vi "SetBox.vi"(8 "error in (no error)":errorcluster, 10 "Box":T1, 11 "FolloWin in":refnum<class "FolloWin.lvclass">) -> (0 "error out":errorcluster, 3 "FolloWin out":refnum<class "FolloWin.lvclass">)   [LabVIEW 2023, in "FolloWin.lvclass"]
doc: "Sets the box (in screen coordinates) \nThe Box defines the active area of FolloWin, meaning, it will only show the FolloWin window if your mouse cursor is inside the box's boundries."
uses:
  FolloWin.lvclass
  <vilib>/Utility/miscctls.llb/LVRectTypeDef.ctl
  FolloWin.lvclass/FolloWin.ctl
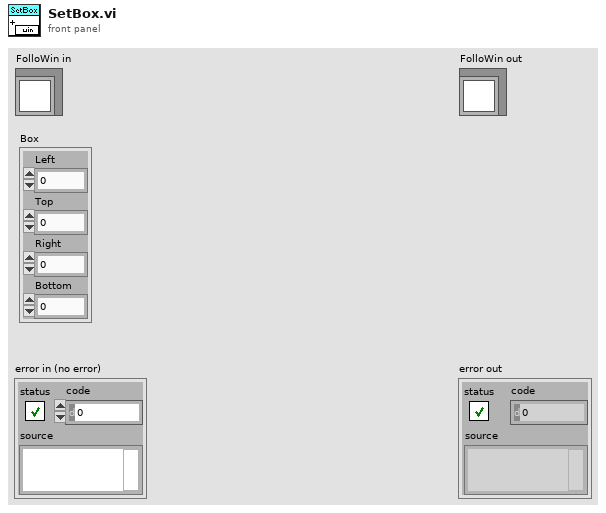
[diagram p1: front panel]
types:
  T1 = typedef "LVRectTypeDef.ctl" = cluster{"Left":i16, "Top":i16, "Right":i16, "Bottom":i16}
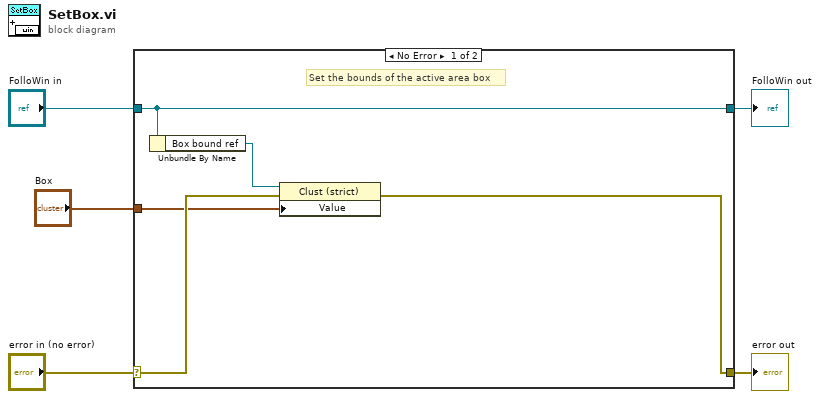
[diagram p0: block diagram]
diagram:
  n1 = case shown="No Error" "error in (no error)" {
    selector: "error in (no error)" -> [w8 w12]
    tunnel: [w7 w12] -> w4
    tunnel: [w10 w11] -> w2
    tunnel: "FolloWin in" -> [w10 w11]
    tunnel: "Box" -> [w6 _]
    frame No Error {
      # "Set the bounds of the active area box"
      n2 = Unbundle By Name(w10) -> ("Box bound ref"=w9:refnum<vi>)
      n3 = property on="Property Node" class="Clust (strict)"(reference=w9, error in=w8, "Value"=w6) -> (error out=w7:errorcluster)  [unwired: 1 out]
    }
    frame Error {
    }
  }
  "error out" <- w4
  "FolloWin out" <- w2
